vi "Read Channel Functions.vi"(8 "error in (no error)":errorcluster, 11 "Generic Data Acquisition in":refnum<class "Generic Data Acquisition.lvclass">) -> (0 "error out":errorcluster, 2 "Channel Functions":i8[](array[numeric]), 3 "Generic Data Acquisition out":refnum<class "Generic Data Acquisition.lvclass">)   [LabVIEW 2014, in "Generic Data Acquisition.lvlib" / "Generic Data Acquisition.lvclass"]
uses:
  Generic Data Acquisition.lvclass
  Generic Data Acquisition.lvclass/Generic Data Acquisition.ctl
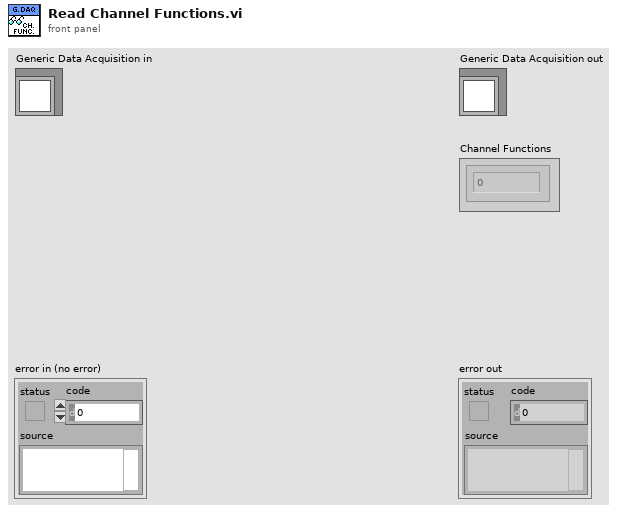
[diagram p1: front panel]
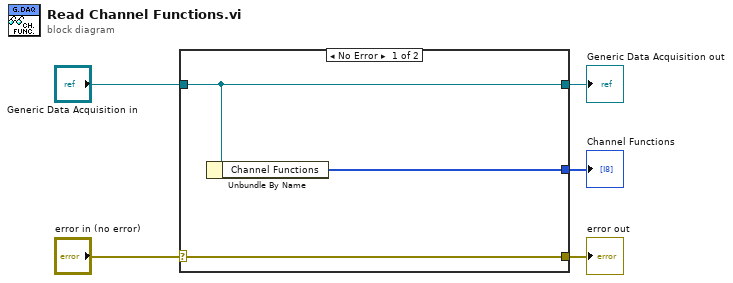
[diagram p0: block diagram]
diagram:
  n1 = case shown="No Error" "error in (no error)" {
    selector: "error in (no error)" -> [w8 w9]
    tunnel: [w8 w9] -> w4
    tunnel: [w7 w10] -> w2
    tunnel: "Generic Data Acquisition in" -> [w7 w10]
    tunnel: [w6 _] -> w1
    frame No Error {
      n2 = Unbundle By Name(w7) -> ("Channel Functions"=w6:i8[])
    }
    frame Error {
    }
  }
  "error out" <- w4
  "Generic Data Acquisition out" <- w2
  "Channel Functions" <- w1
